vi "ACC_LabVIEW_Read.vi"(0 "DeviceReferenceIn":cluster{"ID":u32}, 2 "Propname":string, 3 "return data string buffer size (Byte)":u32, 4 "#of expected Elements in \"Acc_Data_Out\"":u32=1000, 5 "error in (no error)":errorcluster, 7 "return error strings buffer size (Byte)":u32=500, 8 "VirtAcc":i32, 9 "Acc_Para_In":T1[](array[typedef])) -> (14 "DeviceReferenceOut":cluster{"ID":u32}, 15 "Acc_Data_Out":T1[](array[typedef]), 17 "LV_TimeStamp":T4, 18 "EFICD":T3, 19 "error out":errorcluster)   [LabVIEW 2014, in "ACC_LabVIEW.lvlib"]
doc: "Perform a \"read\" inside the GSI - accelerator control system."
uses:
  ACC_LabVIEW.lvlib
  ACC_LabVIEW_Container.ctl
  ACC_LabVIEW_DataTypes.ctl
  lib/ACC_Interface_Wrapper.dll
panel:
  in  "AccData Container":T1={"Data Type"=enum."UByte (8Bit int unsigned)", "String"="", "Double"=0.0}
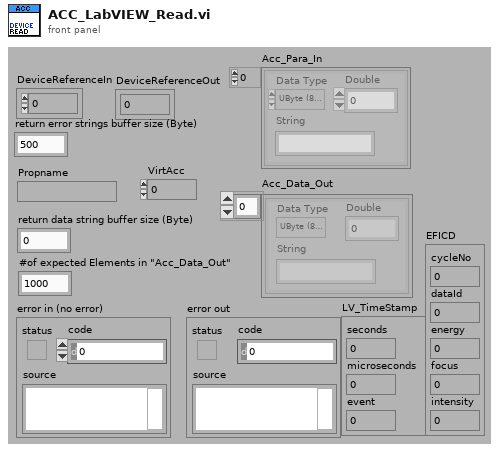
[diagram p1: front panel]
types:
  T1 = typedef "ACC_LabVIEW.lvlib/ACC_LabVIEW_Container.ctl" = cluster{"Data Type":T2, "String":string, "Double":dbl}
  T2 = typedef "ACC_LabVIEW.lvlib/ACC_LabVIEW_DataTypes.ctl" = enum16{"SByte (8Bit Int signed)", "UByte (8Bit int unsigned)", "SWord (16Bit Int signed)", "UWord (16Bit Int unsigned)", "SLong (32Bit Int signed)", "ULong (32Bit Int unsigned)", "Float32 (float)", "Float64 (double)", "String"}
  T3 = cluster{"cycleNo":u32, "dataId":u32, "energy":u32, "focus":u32, "intensity":u32}
  T4 = cluster{"seconds":u32, "microseconds":u32, "event":u32}
  T5 = cluster{"LV_TimeStamp[0]":u32, "LV_TimeStamp[1]":u32, "LV_TimeStamp[2]":u32}
  T6 = cluster{"LV_EFICD[0]":u32, "LV_EFICD[1]":u32, "LV_EFICD[2]":u32, "LV_EFICD[3]":u32, "LV_EFICD[4]":u32}
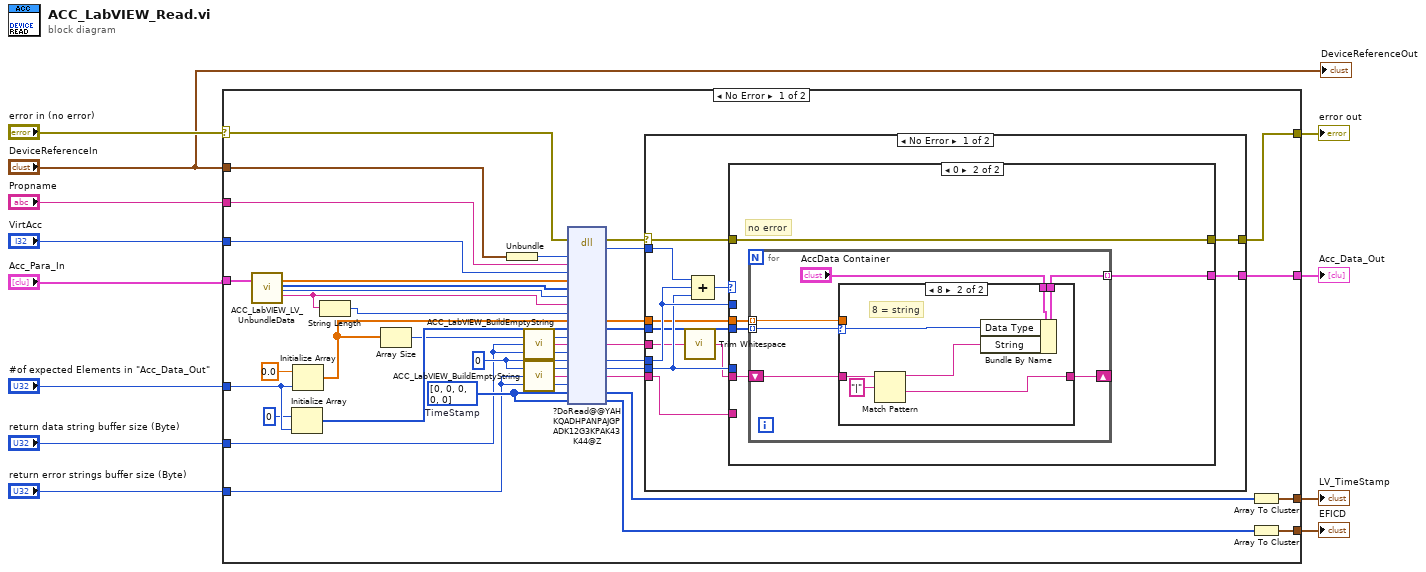
[diagram p0: block diagram]
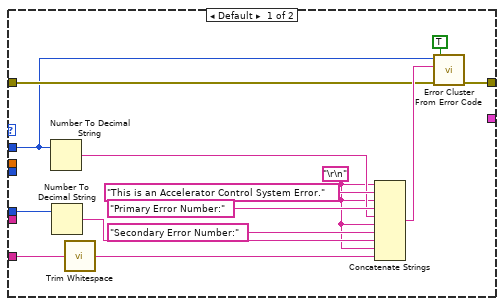
[diagram p2: hidden frame]
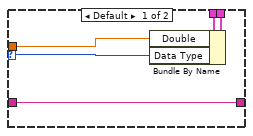
[diagram p3: hidden frame]
diagram:
  n1 = case shown="No Error" "error in (no error)" {
    selector: "error in (no error)" -> [w36 w100]
    tunnel: "Propname" -> [w42 _]
    tunnel: "return data string buffer size (Byte)" -> [w13 _]
    tunnel: "#of expected Elements in \"Acc_Data_Out\"" -> [w48 _]
    tunnel: "VirtAcc" -> [w41 _]
    tunnel: [w47 w100] -> w8
    tunnel: [w46 _] -> w7
    tunnel: [w44 _] -> w5
    tunnel: [w43 _] -> w4
    tunnel: "Acc_Para_In" -> [w19 _]
    tunnel: "DeviceReferenceIn" -> [w16 _]
    tunnel: "return error strings buffer size (Byte)" -> [w14 _]
    frame No Error {
      w33 = u32[] [0, 0, 0, 0, 0]  # TimeStamp
      w35 = u32 0 ("no input, only output")
      n2 = call "ACC_LabVIEW_LV_UnbundleData.vi"("Acc_Data_In"=w19) -> ("LV_double_array"=w22:dbl[], "LV_types"=w21:i32[], "Length"=w20:i32, "Data-String"=w18:string)  [unwired: 15 in]
      n3 = Initialize Array(0, w48) -> (w39:i32[])
      n4 = Initialize Array(0.0, w48) -> (w40:dbl[])
      n5 = String Length(string=w18) -> (length=w17:i32)
      n6 = Array Size(array=w40) -> (size(s)=w38:i32)
      n7 = Unbundle(w16) -> ("ID"=w15:u32)
      n8 = call "ACC_LabVIEW_BuildEmptyString.vi"("Length"=w13) -> ("String"=w37:string)
      n9 = call "ACC_LabVIEW_BuildEmptyString.vi"("Length"=w14) -> ("String"=w34:string)
      n10 = dll-call lib="D:/Git/CS-framework/CSinstr.lib/ACC_LabVIEW_Interface/lib/ACC_Interface_Wrapper.dll" fn="?DoRead@@YAHKQADHPANPAJGPADK12G3KPAK43K44@Z"(error in=w36, "DeviceHandle"=w15, "LV_propname"=w42, "LV_VirtAcc"=w41, "LV_para"=w22, "LV_para_types"=w21, "LV_para_Size"=w20, "LV_para_string"=w18, "LV_para_string_Size"=w17, "LV_data"=w40, "LV_data_types"=w39, "LV_data_Size"=w38, "LV_data_string"=w37, "LV_data_string_Size"=w13, "ErrPrimStat"=w35, "ErrSecStat"=w35, "ErrorMSG"=w34, "ErrorMSG_Size"=w14, "LV_TimeStamp"=w33, "LV_EFICD"=w33) -> (error out=w32:errorcluster, "ErrorPrimState"=w31:i32, "LV_data"=w24:dbl[], "LV_data_types"=w23:i32[], "LV_data_string"=w30:string, "ErrPrimStat"=w28:u32, "ErrSecStat"=w27:u32, "ErrorMSG"=w29:string, "LV_TimeStamp"=w26:u32[], "LV_EFICD"=w25:u32[])  [unwired: 13 in, 1 out]
      n11 = case shown="No Error" w32 {
        selector: w32 -> [w59 w99]
        tunnel: w31 -> [w61 _]
        tunnel: [w56 w99] -> w47
        tunnel: w29 -> [w54 _]
        tunnel: w28 -> [w58 _]
        tunnel: w27 -> [w57 _]
        tunnel: w30 -> [w53 _]
        tunnel: [w55 _] -> w46
        tunnel: w24 -> [w51 _]
        tunnel: w23 -> [w50 _]
        frame No Error {
          n12 = call <vilib>:"Trim Whitespace.vi"("string"=w53) -> ("trimmed string"=w52:string)  [unwired: 1 in]
          n13 = Compound Arithmetic op=ADD(w61, w58, w57) -> (w60:u32)
          n14 = case shown="0" w60 {
            tunnel: w52 -> [_ w79]
            tunnel: w59 -> [w65 w80]
            tunnel: w58 -> [w63 _]
            tunnel: w57 -> [w75 _]
            tunnel: [w64 w80] -> w56
            tunnel: [_ w78] -> w55
            tunnel: w54 -> [w69 _]
            tunnel: w51 -> [_ w77]
            tunnel: w50 -> [_ w76]
            frame Default {
              w67 = "\r\n"
              n15 = Number To Decimal String(number=w63) -> (decimal integer string=w72:string)  [unwired: 1 in]
              n16 = Number To Decimal String(number=w75) -> (decimal integer string=w70:string)  [unwired: 1 in]
              n17 = call <vilib>:"Trim Whitespace.vi"("string"=w69) -> ("trimmed string"=w68:string)  [unwired: 1 in]
              n18 = Concatenate Strings(w67, "This is an Accelerator Control System Error.", w67, "Primary Error Number:", w72, w67, "Secondary Error Number:", w70, w67, w68) -> (w66:string)
              n19 = call <vilib>:"Error Cluster From Error Code.vi"("show call chain? (False)"=TRUE, "error in (no error)"=w65, "error message (\"\")"=w66, "error code (0)"=w63) -> ("error out"=w64:errorcluster)  [unwired: 5 in]
            }
            frame 0 {
              # "no error"
              n20 = for {
                shift-right: [w84] -> _
                shift-left: w79 -> [w85]
                tunnel: [w83] -> w78 mode=indexing
                tunnel: w77 -> [w82] mode=indexing
                tunnel: w76 -> [w81] mode=indexing
                n21 = case shown="8" w81 {
                  selector: w81 -> [w90 w97]
                  tunnel: "AccData Container" -> [w89 w98]
                  tunnel: w85 -> [w91 w96]
                  tunnel: [w91 w94] -> w84
                  tunnel: [w88 w92] -> w83
                  tunnel: w82 -> [w87 _]
                  frame Default {
                    n22 = Bundle By Name(cluster=w89, "Double"=w87, "Data Type"=w90) -> (w88:T1)
                  }
                  frame 8 {
                    # "8 = string"
                    n23 = Match Pattern(string=w96, regular expression="|") -> (before substring=w93:string, after substring=w94:string)  [unwired: 1 in, 2 out]
                    n24 = Bundle By Name(cluster=w98, "Data Type"=w97, "String"=w93) -> (w92:T1)
                  }
                }
              }
            }
          }
        }
        frame Error {
        }
      }
      n25 = Array To Cluster(array=w26) -> (cluster=w44:T5)
      n26 = Array To Cluster(array=w25) -> (cluster=w43:T6)
    }
    frame Error {
    }
  }
  "error out" <- w8
  "Acc_Data_Out" <- w7
  "LV_TimeStamp" <- w5
  "EFICD" <- w4
  "DeviceReferenceOut" <- "DeviceReferenceIn"
